vi "Get Wind Dir Str V.vi"(8 "error in (no error)":errorcluster, 11 "dirStr":string) -> (0 "error out":errorcluster, 2 "function return":string, 3 "dirStr out":string)   [LabVIEW 2012, in "VantagePro.lvlib"]
doc: "DllAccess char* _stdcall GetWindDirStr_V(char* dirStr);"
uses:
  VantagePro.lvlib
  VantagePro.dll
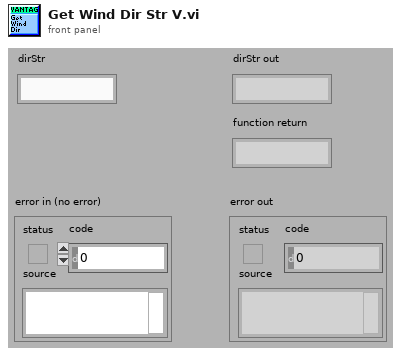
[diagram p1: front panel]
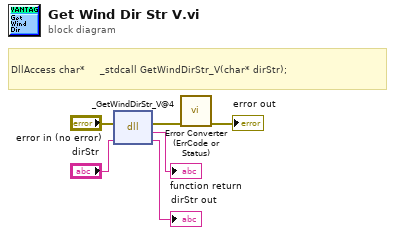
[diagram p0: block diagram]
diagram:
  # "DllAccess char*     _stdcall GetWindDirStr_V(char* dirStr);"
  n1 = dll-call lib="C:/Users/Dimitris/Desktop/BRITE/libs/VantagePro/VantagePro.*" fn="_GetWindDirStr_V@4"(error in="error in (no error)", "dirStr"="dirStr") -> (error out=w2:errorcluster, →"function return":string, "dirStr"=→"dirStr out":string)  [unwired: 2 in, 1 out]
  n2 = call "Error Converter (ErrCode or Status).vi"("error in (no error)"=w2) -> ("error out"=→"error out":errorcluster)  [unwired: 10 in]
